vi "SetPosition.vi"(8 "error in (no error)":errorcluster, 10 "position (\"\")":string, 11 "object in":refnum<class "Board.lvclass">) -> (0 "error out":errorcluster, 3 "object out":refnum<class "Board.lvclass">)   [LabVIEW 2020, in "Board.lvclass"]
uses:
  Board.lvclass
  Board.lvclass/Board.ctl
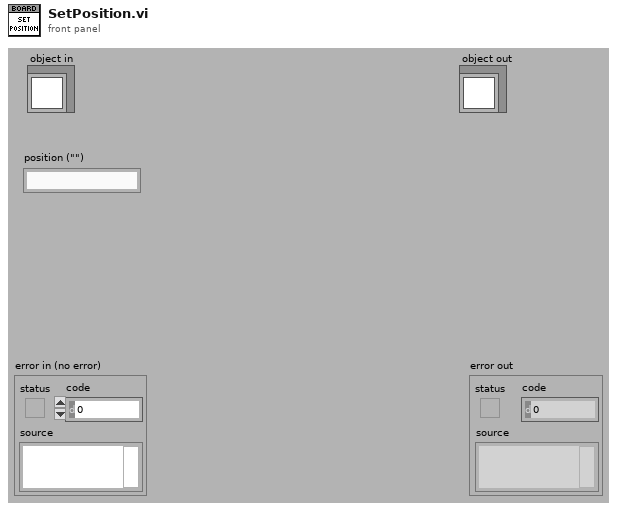
[diagram p1: front panel]
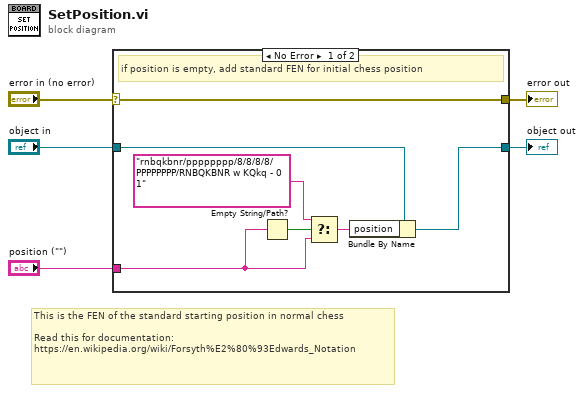
[diagram p0: block diagram]
diagram:
  # "This is the FEN of the standard starting position in normal chess\n\nRead this for documentation:\nhttps://en.wikipedia.org/wiki/Forsyth%E2%80%93Edwards_Notation"
  n1 = case shown="No Error" "error in (no error)" {
    selector: "error in (no error)" -> [w12 w14]
    tunnel: [w12 w14] -> w4
    tunnel: [w10 w13] -> w2
    tunnel: "object in" -> [w11 w13]
    tunnel: "position (\"\")" -> [w7 _]
    frame No Error {
      # "if position is empty, add standard FEN for initial chess position"
      n2 = Empty String/Path?(string/path=w7) -> (empty?=w9:bool)
      n3 = Select(t="rnbqkbnr/pppppppp/8/8/8/8/PPPPPPPP/RNBQKBNR w KQkq - 0 1" ("board"), s=w9, f=w7) -> (s? t:f=w6:string)
      n4 = Bundle By Name(cluster=w11, "position"=w6) -> (w10:refnum<class "Board.lvclass">)
    }
    frame Error {
    }
  }
  "error out" <- w4
  "object out" <- w2
